vi "LatestInstallers.vi"(7 "Minutes to wait":u32, 8 "error in":errorcluster, 9 "path to search latest folder CSDS":path, 10 "path to search latest folder LVMD":path, 11 "Latest installers":T3 {"Machine Name" items=["Machine-01", "Machine-02", "Machine-03", "Machine-04", "Machine-05", "Machine-06", "Machine-07", "Machine-08", "Machine-09", "Machine-10", "Machine-11", "Machine-12", "Machine-13", "Machine-14", "Machine-15", "Machine-16"]; "Branch-CSDS" items=["R3-Trunk", "R2-VI Main", "R2-SB", "R2-SD", "R2-Trunk"]; "Branch-LVMD" items=["R3-Trunk", "R2-VI Main", "R2-SB", "R2-SD", "R2-Trunk"]}) -> (0 "error out":errorcluster)   [LabVIEW 2013]
uses:
  ControlLatestInstall.ctl
  ControlBranchName.ctl
  MachineNames.ctl
  <vilib>/Utility/config.llb/Read Key (String).vi
  <vilib>/Utility/config.llb/NI_LVConfig.lvlib
panel:
  out "Branch-LVMD":T1 items=["R2-Releases-LVMD[NI]", "R2-Releases-MCC[NI]"]
  out "Branch-CSDS":T1 items=["R2-Releases-LVMD[NI]", "R2-Releases-MCC[NI]"]
  out "Machine Name":T2=3 items=["Machine-01", "Machine-02", "Machine-03", "Machine-04", "Machine-05", "Machine-06", "Machine-07", "Machine-08", "Machine-09", "Machine-10", "Machine-11", "Machine-12", "Machine-13", "Machine-14", "Machine-15", "Machine-16"]
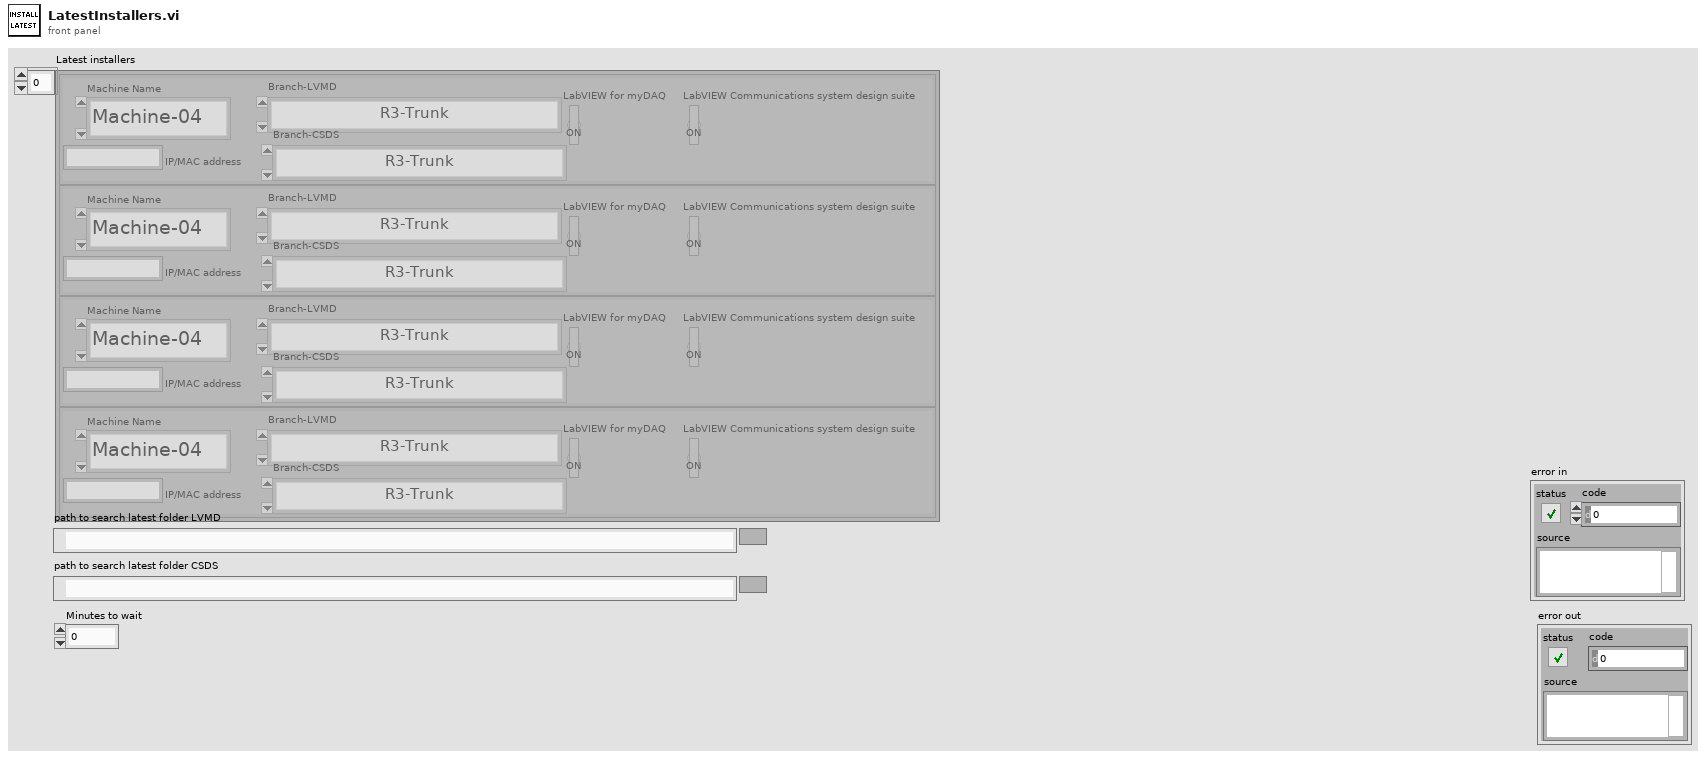
[diagram p1: front panel]
types:
  T1 = typedef "ControlBranchName.ctl" = u16
  T2 = typedef "MachineNames.ctl" = u16
  T3 = typedef "ControlLatestInstall.ctl" = cluster{"Branch-LVMD":T1, "LabVIEW for myDAQ":bool, "LabVIEW Communications system design suite":bool, "IP/MAC address":string, "Branch-CSDS":T1, "Machine Name":T2}[]
  T4 = typedef "NI_LVConfig.lvlib/Config Data RefNum.ctl" = refnum<k1>
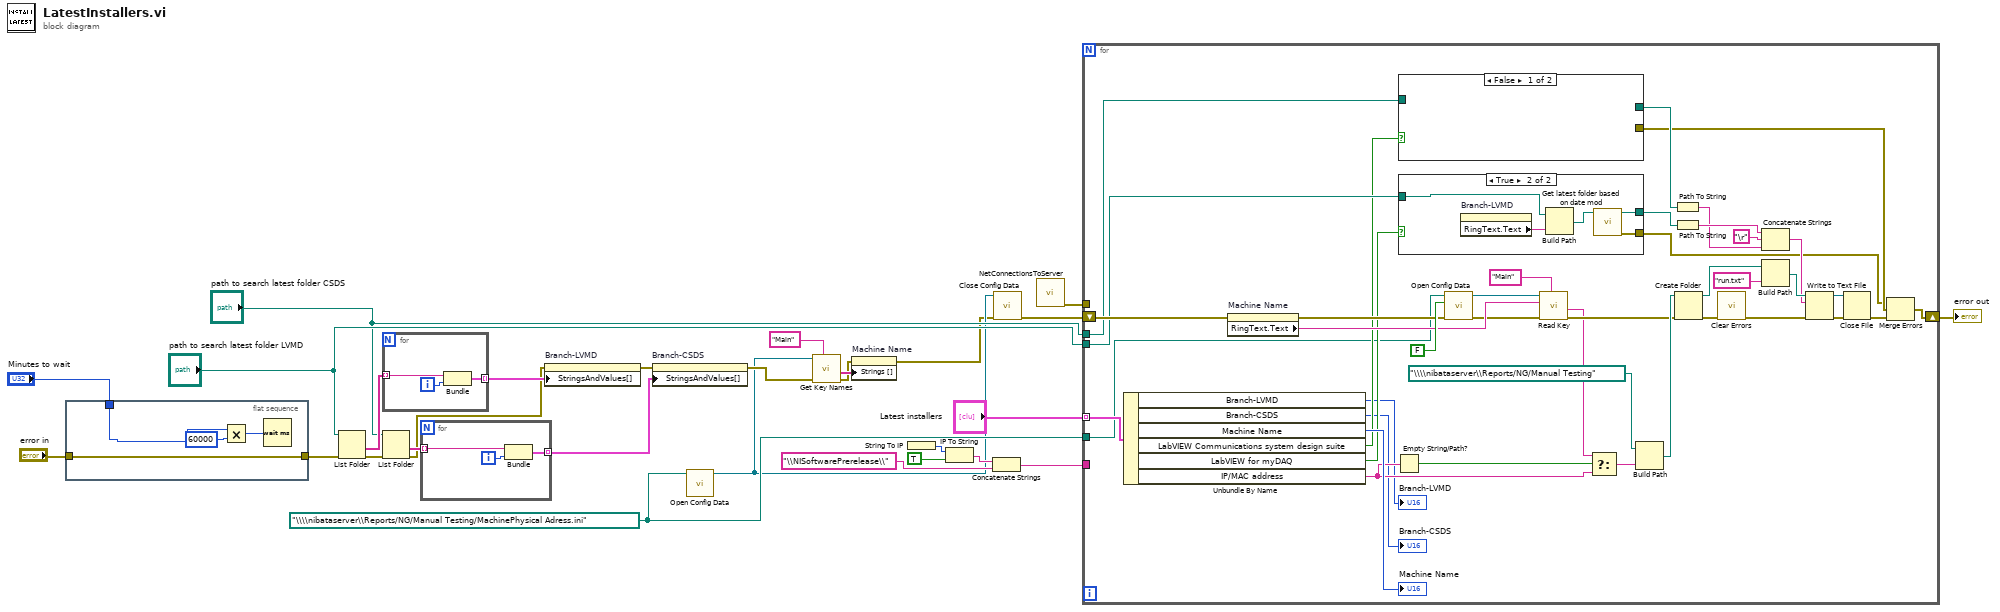
[diagram p0: block diagram]
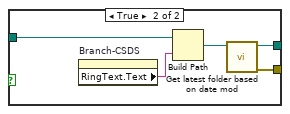
[diagram p2: hidden frame]
diagram:
  w13 = path "\\\\nibataserver\\Reports/NG/Manual Testing/MachinePhysical Adress.ini" ("configuration file path")
  n1 = flat-sequence {
    tunnel: "error in" -> [w32]
    tunnel: [w32] -> w2
    tunnel: "Minutes to wait" -> [w29]
    frame #0 {
      n2 = Multiply(x=w29, y=u32 60000) -> (x*y=w31:u32)
      n3 = Wait (ms)(milliseconds to wait=w31) -> ()  [unwired: 1 out]
    }
  }
  n4 = List Folder(path="path to search latest folder LVMD", error in=w2) -> (folder names=w20:string[], error out=w5:errorcluster)  [unwired: 2 in, 2 out]
  n5 = for {
    tunnel: w20 -> [w35] mode=indexing
    tunnel: [w33] -> w16 mode=indexing
    i -> [w34]
    n6 = Bundle(w35, w34) -> (w33:cluster{string, i32})  [unwired: 1 in]
  }
  n7 = List Folder(path="path to search latest folder CSDS", error in=w5) -> (folder names=w18:string[], error out=w4:errorcluster)  [unwired: 2 in, 2 out]
  n8 = for {
    tunnel: w18 -> [w38] mode=indexing
    tunnel: [w36] -> w15 mode=indexing
    i -> [w37]
    n9 = Bundle(w38, w37) -> (w36:cluster{string, i32})  [unwired: 1 in]
  }
  n10 = property on="Branch-LVMD" class="Ring (strict)"(error in=w4, "StringsAndValues[]"=w16) -> (error out=w14:errorcluster)  [unwired: 1 in, 1 out]
  n11 = property on="Branch-CSDS" class="Ring (strict)"(error in=w14, "StringsAndValues[]"=w15) -> (error out=w10:errorcluster)  [unwired: 1 in, 1 out]
  n12 = call <vilib>:"Open Config Data.vi"("configuration file path"=w13) -> ("refnum"=w8:T4)  [unwired: 8 in, 2 out]
  n13 = call <vilib>:"Get Key Names.vi"("section"="Main", "error in (no error)"=w10, "refnum"=w8) -> ("error out"=w11:errorcluster, "key names"=w12:string[])  [unwired: 5 in, 2 out]
  n14 = property on="Machine Name" class="Ring (strict)"(error in=w11, "Strings []"=w12) -> (error out=w7:errorcluster)  [unwired: 1 in, 1 out]
  n15 = String To IP() -> (0:w26:u32)  [unwired: 1 in]
  n16 = IP To String(1:TRUE ("dot notation? (F)"), 2:w26) -> (0:w25:string)
  n17 = Concatenate Strings(w25, "\\NISoftwarePrerelease\\") -> (w23:string)
  n18 = call <vilib>:"Close Config Data.vi"("error in (no error)"=w7, "refnum"=w8) -> ("error out"=w6:errorcluster)  [unwired: 8 in, 1 out]
  n19 = call "NetConnectionsToServer.vi"() -> ("error out"=w21:errorcluster)  [unwired: 11 in]
  n20 = for {
    tunnel: "Latest installers" -> [w77] mode=indexing
    tunnel: w23 -> [_]
    shift-right: [w52] -> w22
    shift-left: w6 -> [w56]
    tunnel: w21 -> [_]
    tunnel: "path to search latest folder LVMD" -> [w46]
    tunnel: "path to search latest folder CSDS" -> [w45]
    tunnel: w13 -> [w39]
    n21 = Unbundle By Name(w77) -> ("Branch-LVMD"=→"Branch-LVMD":T1, "Branch-CSDS"=→"Branch-CSDS":T1, "Machine Name"=→"Machine Name":T2, "LabVIEW Communications system design suite"=w44:bool, "LabVIEW for myDAQ"=w43:bool, "IP/MAC address"=w48:string)
    n22 = property on="Machine Name" class="Ring (strict)"(error in=w56) -> (error out=w58:errorcluster, "RingText.Text"=w68:string)  [unwired: 1 in, 1 out]
    n23 = Empty String/Path?(string/path=w48) -> (empty?=w50:bool)
    n24 = case shown="False" w44 {
      tunnel: [_ w83] -> w62
      tunnel: [_ w82] -> w55
      tunnel: w45 -> [_ w80]
      frame False {
      }
      frame True {
        n25 = property on="Branch-CSDS" class="Ring (strict)"() -> ("RingText.Text"=w79:string)  [unwired: 2 in, 2 out]
        n26 = Build Path(base path=w80, name or relative path=w79) -> (appended path=w81:path)
        n27 = call "Get latest folder based on date mod.vi"("path"=w81) -> ("error out"=w82:errorcluster, "appended path"=w83:path)  [unwired: 9 in]
      }
    }
    n28 = case shown="True" w43 {
      tunnel: [_ w88] -> w66
      tunnel: [_ w87] -> w54
      tunnel: w46 -> [_ w86]
      frame False {
      }
      frame True {
        n29 = property on="Branch-LVMD" class="Ring (strict)"() -> ("RingText.Text"=w84:string)  [unwired: 2 in, 2 out]
        n30 = Build Path(base path=w86, name or relative path=w84) -> (appended path=w85:path)
        n31 = call "Get latest folder based on date mod.vi"("path"=w85) -> ("error out"=w87:errorcluster, "appended path"=w88:path)  [unwired: 9 in]
      }
    }
    n32 = call <vilib>:"Open Config Data.vi"("error in (no error)"=w58, "create file if necessary (T)"=FALSE, "configuration file path"=w39) -> ("error out"=w59:errorcluster, "refnum"=w40:T4)  [unwired: 6 in, 1 out]
    n33 = call-poly <vilib>:"Read Key.vi"("section"="Main", "error in (no error)"=w59, "key"=w68, "refnum"=w40) -> ("error out"=w60:errorcluster, "value"=w49:string)  [unwired: 4 in, 2 out]
    n34 = Select(t=w49, s=w50, f=w48) -> (s? t:f=w47:string)
    n35 = Build Path(base path=path "\\\\nibataserver\\Reports/NG/Manual Testing", name or relative path=w47) -> (appended path=w74:path)
    n36 = Path To String(path=w62) -> (string=w63:string)
    n37 = Path To String(path=w66) -> (string=w65:string)
    n38 = Create Folder(path (use dialog)=w74, error in=w60) -> (created path=w73:path, error out=w72:errorcluster)  [unwired: 1 in, 1 out]
    n39 = call <vilib>:"Clear Errors.vi"("error in (no error)"=w72) -> ("error out"=w71:errorcluster)  [unwired: 6 in]
    n40 = Concatenate Strings(w65, "\r", w63) -> (w61:string)
    n41 = Build Path(base path=w73, name or relative path="run.txt") -> (appended path=w75:path)
    n42 = Write to Text File(file (use dialog)=w75, text=w61, error in=w71) -> (refnum out=w67:refnum<file>, error out=w57:errorcluster)  [unwired: 1 in, 1 out]
    n43 = Close File(refnum=w67, error in=w57) -> (error out=w53:errorcluster)  [unwired: 1 out]
    n44 = Merge Errors(w54, w55, w53) -> (w52:errorcluster)
  }
  "error out" <- w22
